vi "CSV_Setup_Data.vi"() -> ()   [LabVIEW 2019]
uses:
  controls/Data.ctl
  <vilib>/userdefined/High Color/IMAQdx.ctl
  <vilib>/vision/Image Controls.llb/IMAQ Image.ctl
  <vilib>/Utility/file.llb/Write Delimited Spreadsheet (string).vi
panel:
  in  "Image path":string
  in  "Sample Name":string
  in  "input cluster":T1={"L16 Linear Actuator"="", "XE 1000 Pump"="", "Camera1"="", "Camera2"="", "Camera1_IMG"=refnum, "Camera2_IMG"=refnum, "Img_Capt"=FALSE, "Actuator"=FALSE, "Pump"=FALSE, "Cam 1"=FALSE, "Cam 2"=FALSE, "Empty_Refill"=FALSE, "Crop"=FALSE, "Light intensity"=100, "Exposure Time"=1000.0, "Sample Name"="Test Sample", "Operator"="MRJ", "Calibration 1"=path "C:/Users/au540322/Desktop/IHS_Project/images/Debris/Debris_0/Debris_0_2019_06_01-23-32-49-686.PNG", "Calibration 2"=path "C:/Users/au540322/Desktop/IHS_Project/images/Debris/Debris_0/Debris_0_2019_06_01-23-32-49-686.PNG", "Framerate"=1, "Timeout Sample"=50, "Collection date"="MRJ", "Cam 1 queue"=refnum, "Cam 2 queue"=refnum, "Sample size threshold"=1, "Empty start"=1, "Command"="MRJ", "Calibration Image 1"=refnum, "Calibration Image 2"=refnum, "Original Image 1"=refnum, "Original Image 2"=refnum, "Processing Image 1"=refnum, "Processing Image 2"=refnum, "Object Image 1"=refnum, "Object Image 2"=refnum, "Cam 1 - save queue"=refnum, "Cam 2 - save queue"=refnum, "Station"="", "Species Name"="", "Other Notes"="", "Aperture"=enum."Item 0", "Image Process Queue Size"=10, "Image Save Queue Size"=1, "Overload threshold"=500, "Max Framerate"=100, "Blue Plane Image"=refnum, "Subtract Image"=refnum, "Binary Image"=refnum} {"Max Framerate" min=1; "Overload threshold" min=1; "Image Save Queue Size" min=1; "Image Process Queue Size" min=1; "Empty start" min=1; "Sample size threshold" min=1; "Framerate" min=1; "Light intensity" scale=0.0..100.0}
  in  "file path (dialog if empty)":path
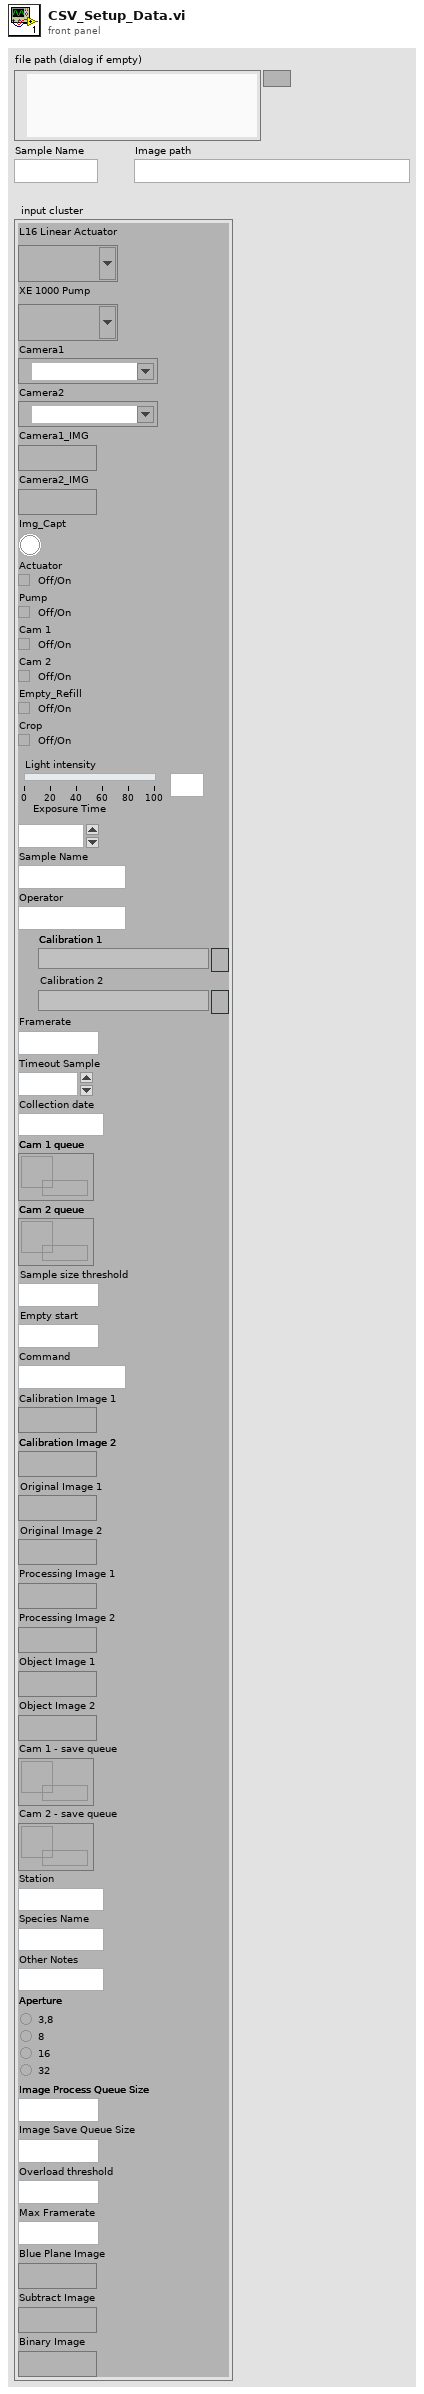
[diagram p1: front panel]
types:
  T1 = typedef "Data.ctl" = cluster{"L16 Linear Actuator":refnum<visa-resource-name>, "XE 1000 Pump":refnum<visa-resource-name>, "Camera1":T2, "Camera2":T2, "Camera1_IMG":T3, "Camera2_IMG":T3, "Img_Capt":bool, "Actuator":bool, "Pump":bool, "Cam 1":bool, "Cam 2":bool, "Empty_Refill":bool, "Crop":bool, "Light intensity":i32, "Exposure Time":dbl, "Sample Name":string, "Operator":string, "Calibration 1":path, "Calibration 2":path, "Framerate":i32, "Timeout Sample":i32, "Collection date":string, "Cam 1 queue":refnum<queue>, "Cam 2 queue":refnum<queue>, "Sample size threshold":i32, "Empty start":u32, "Command":string, "Calibration Image 1":T3, "Calibration Image 2":T3, "Original Image 1":T3, "Original Image 2":T3, "Processing Image 1":T3, "Processing Image 2":T3, "Object Image 1":T3, "Object Image 2":T3, "Cam 1 - save queue":refnum<queue>, "Cam 2 - save queue":refnum<queue>, "Station":string, "Species Name":string, "Other Notes":string, "Aperture":enum32{"Item 0", "Item 1", "Item 2", "Item 3"}, "Image Process Queue Size":i32, "Image Save Queue Size":i32, "Overload threshold":i32, "Max Framerate":i32, "Blue Plane Image":T3, "Subtract Image":T3, "Binary Image":T3}
  T2 = typedef "IMAQdx.ctl" = refnum<k21>
  T3 = typedef "IMAQ Image.ctl" = refnum<image>
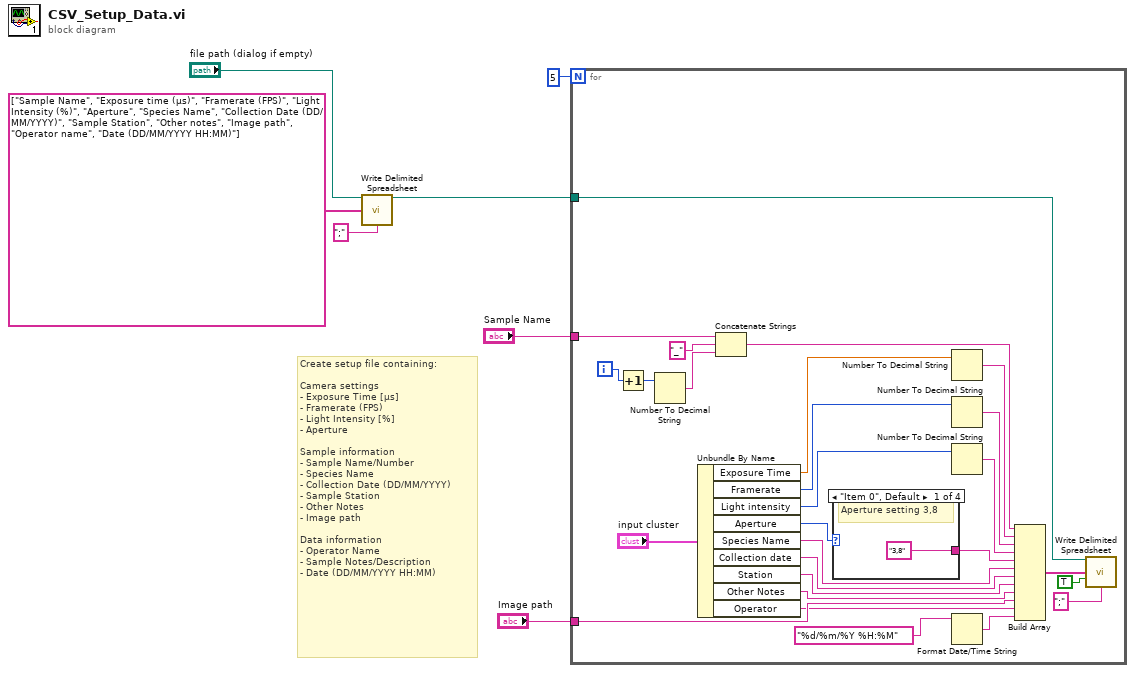
[diagram p0: block diagram]
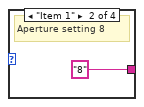
[diagram p2: hidden frame]
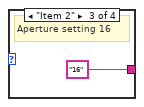
[diagram p3: hidden frame]
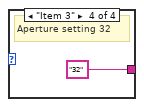
[diagram p4: hidden frame]
diagram:
  # "Create setup file containing:\n\nCamera settings\n- Exposure Time [µs]\n- Framerate (FPS)\n- Light Intensity [%]\n- Aperture\n\nSample information\n- Sample Name/Number\n- Species Name\n- Collection Date (DD/MM/YYYY)\n- Sample Station\n- Other Notes\n- Image path\n\nData information\n- Operator Name\n- Sample Notes/Description\n- Date (DD/MM/YYYY HH:MM)"
  n1 = call-poly <vilib>:"Write Delimited Spreadsheet.vi"("file path (dialog if empty)"="file path (dialog if empty)", "1D data"=string[] ["Sample Name", "Exposure time (µs)", "Framerate (FPS)", "Light Intensity (%)", "Aperture", "Species Name", "Collection Date (DD/MM/YYYY)", "Sample Station", "Other notes", "Image path", "Operator name", "Date (DD/MM/YYYY HH:MM)"], "delimiter (\\t)"=";" ("delimiter (\\t)")) -> ("new file path (Not A Path if cancelled)"=w6:path)  [unwired: 11 in, 1 out]
  n2 = for {
    N: 5 -> [_]
    tunnel: w6 -> [w29]
    tunnel: "Sample Name" -> [w18]
    tunnel: "Image path" -> [w9]
    i -> [w17]
    n3 = Increment(x=w17) -> (x+1=w13:i32)
    n4 = Number To Decimal String(number=w13) -> (decimal integer string=w15:string)  [unwired: 1 in]
    n5 = Unbundle By Name("input cluster") -> ("Exposure Time"=w32:dbl, "Framerate"=w31:i32, "Light intensity"=w30:i32, "Aperture"=w11:enum32{"Item 0", "Item 1", "Item 2", "Item 3"}, "Species Name"=w25:string, "Collection date"=w24:string, "Station"=w23:string, "Other Notes"=w22:string, "Operator"=w8:string)
    n6 = Concatenate Strings(w18, "_" ("string"), w15) -> (w14:string)
    n7 = case shown="\"Item 0\", Default" w11 {
      tunnel: ["3,8" "8" "16" "32"] -> w10
      frame "Item 0", Default {
        # "Aperture setting 3,8"
      }
      frame "Item 1" {
        # "Aperture setting 8"
      }
      frame "Item 2" {
        # "Aperture setting 16"
      }
      frame "Item 3" {
        # "Aperture setting 32"
      }
    }
    n8 = Number To Decimal String(number=w32) -> (decimal integer string=w28:string)  [unwired: 1 in]
    n9 = Number To Decimal String(number=w31) -> (decimal integer string=w27:string)  [unwired: 1 in]
    n10 = Number To Decimal String(number=w30) -> (decimal integer string=w26:string)  [unwired: 1 in]
    n11 = Format Date/Time String(time format string (%c)="%d/%m/%Y %H:%M") -> (date/time string=w12:string)  [unwired: 2 in]
    n12 = Build Array(w14, w28, w27, w26, w10, w25, w24, w23, w22, w9, w8, w12) -> (w21:string[])
    n13 = call-poly <vilib>:"Write Delimited Spreadsheet.vi"("file path (dialog if empty)"=w29, "1D data"=w21, "append to file? (new file:F)"=TRUE, "delimiter (\\t)"=";" ("delimiter (\\t)")) -> ()  [unwired: 10 in, 2 out]
  }
